vi "STS_Get_Target_Wavelength_Table.vi"(8 "错误输入（无错误）":errorcluster, 11 ".NET引用句柄输入":refnum<k24>) -> (0 "error out":errorcluster, 1 "wavelengths":dbl[](array[numeric]), 3 "引用输出":refnum<k24>)   [LabVIEW 2017]
doc: "Get Rescaled wavelength tabel"
uses:
  D:/test/ILSTS/LV_IL_Sample/DLL/STSProcess.dll
  DLL/STSProcess.dll
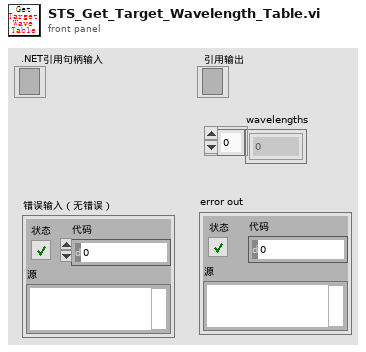
[diagram p1: front panel]
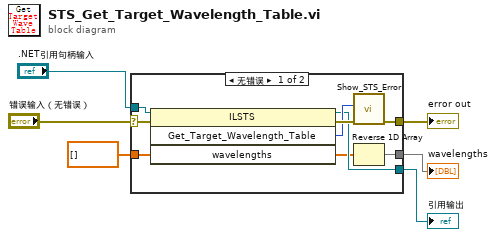
[diagram p0: block diagram]
diagram:
  n1 = case shown="无错误" "错误输入（无错误）" {
    selector: "错误输入（无错误）" -> [w14 w18]
    tunnel: ".NET引用句柄输入" -> [w15 w17]
    tunnel: [w11 w18] -> w4
    tunnel: [w10 w17] -> w3
    tunnel: [w7 w16] -> w2
    tunnel: dbl[] [] ("wavelengths") -> [w9 w16]
    frame No Error {
      n2 = invoke class="ILSTS" method="Get_Target_Wavelength_Table"(reference=w15, error in=w14, "wavelengths"=w9) -> (reference out=w10:refnum<k24>, error out=w13:errorcluster, "Get_Target_Wavelength_Table"=w12:i32, "wavelengths"=w8:dbl[])  [unwired: 1 in]
      n3 = call "Show_STS_Error.vi"("error in (no error)"=w13, "Error"=w12) -> ("error out"=w11:errorcluster)  [unwired: 9 in]
      n4 = Reverse 1D Array(array=w8) -> (reversed array=w7:dbl[])
    }
    frame Error {
    }
  }
  "error out" <- w4
  "引用输出" <- w3
  "wavelengths" <- w2
